vi "array_referencing.vi"() -> ()   [LabVIEW 2016]
uses:
  Type_Defs/Analog_In.ctl
panel:
  out "Array 3":u16[][](array[numeric])
  out "size(s)":i32
  out "Array 2":u16[](array[numeric])
  in  "Array":T1[](array[typedef])
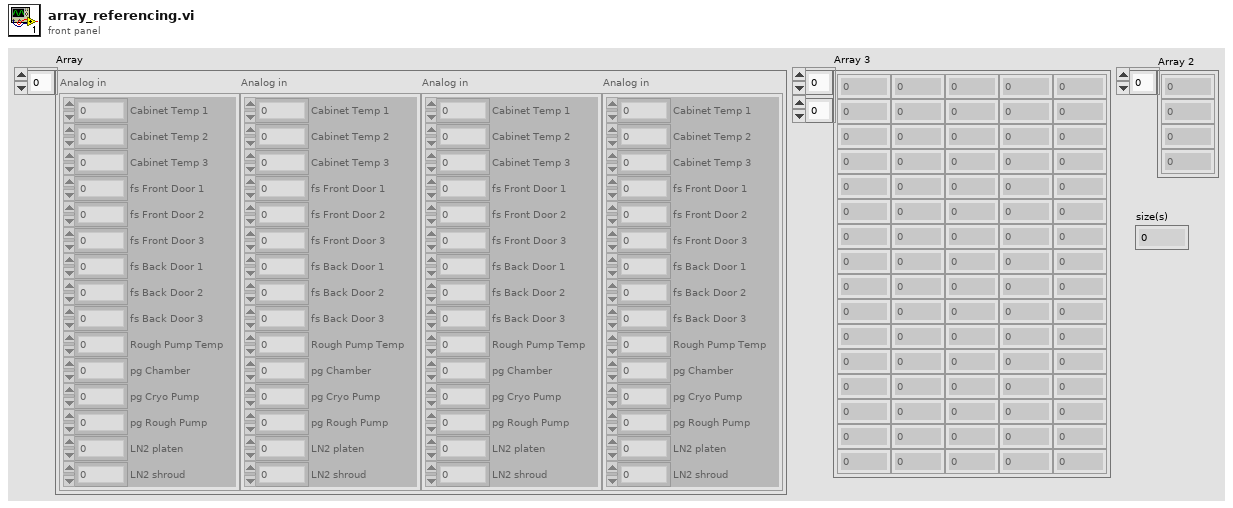
[diagram p1: front panel]
types:
  T1 = typedef "Analog_In.ctl" = cluster{"Cabinet Temp 1":u16, "Cabinet Temp 2":u16, "Cabinet Temp 3":u16, "fs Front Door 1":u16, "fs Front Door 2":u16, "fs Front Door 3":u16, "fs Back Door 1":u16, "fs Back Door 2":u16, "fs Back Door 3":u16, "Rough Pump Temp":u16, "pg Chamber":u16, "pg Cryo Pump":u16, "pg Rough Pump":u16, "LN2 platen":u16, "LN2 shroud":u16}
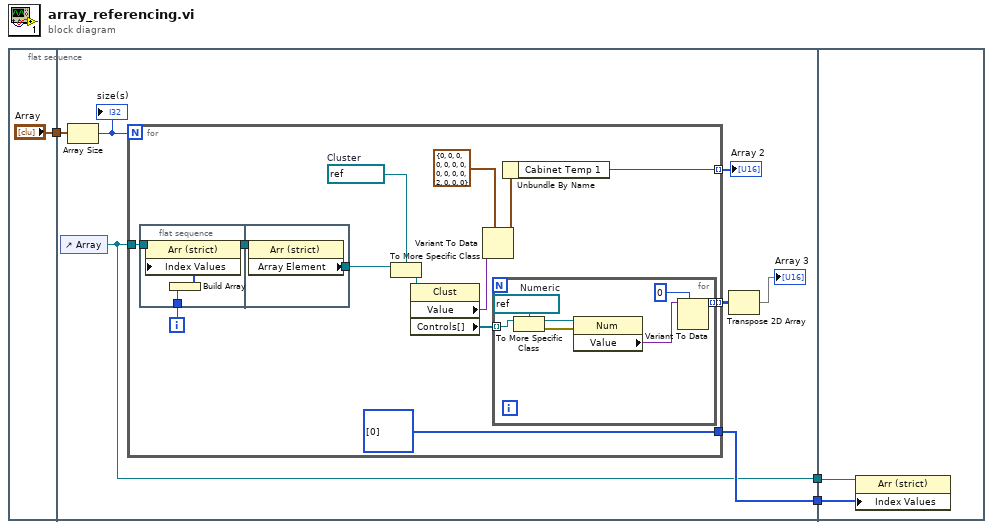
[diagram p0: block diagram]
diagram:
  n1 = flat-sequence {
    tunnel: ["Array"] -> w1
    tunnel: [w9] -> w3
    tunnel: [w8] -> w2
    tunnel: w1 -> [w5]
    tunnel: w3 -> [w38]
    tunnel: w2 -> [w39]
    frame #0 {
    }
    frame #1 {
      n2 = control-ref of="Array"() -> (w8:refnum<vi>)
      n3 = Array Size(array=w5) -> (size(s)=w11:i32)
      "size(s)" <- w11
      n4 = for {
        N: w11 -> [_]
        tunnel: w8 -> [w24]
        tunnel: [w17] -> w10 mode=indexing
        tunnel: [u32[] [0] ("Index Values")] -> w9
        tunnel: [w14] -> w7 mode=indexing
        i -> [w23]
        w19 = refnum<vi> refnum  # Cluster
        n5 = flat-sequence {
          tunnel: w24 -> [w28]
          tunnel: w23 -> [w27]
          tunnel: [w25] -> w13
          tunnel: w13 -> [w30]
          tunnel: [w29] -> w12
          frame #0 {
            n6 = Build Array(w27) -> (w26:i32[])
            n7 = property class="Arr (strict)"(reference=w28, "Index Values"=w26) -> (reference out=w25:refnum<vi>)  [unwired: 1 in, 1 out]
          }
          frame #1 {
            n8 = property class="Arr (strict)"(reference=w30) -> ("Array Element"=w29:refnum<vi>)  [unwired: 1 in, 2 out]
          }
        }
        n9 = To More Specific Class(target class=w19, reference=w12) -> (specific class reference=w20:refnum<vi>)  [unwired: 1 in, 1 out]
        n10 = property class="Clust"(reference=w20) -> ("Value"=w22:variant, "Controls[]"=w15:refnum<vi>[])  [unwired: 1 in, 2 out]
        n11 = Variant To Data(type=T1 {"Cabinet Temp 1"=0, "Cabinet Temp 2"=0, "Cabinet Temp 3"=0, "fs Front Door 1"=0, "fs Front Door 2"=0, "fs Front Door 3"=0, "fs Back Door 1"=0, "fs Back Door 2"=0, "fs Back Door 3"=0, "Rough Pump Temp"=0, "pg Chamber"=0, "pg Cryo Pump"=2, "pg Rough Pump"=0, "LN2 platen"=0, "LN2 shroud"=0} ("Analog in 2"), Variant=w22) -> (data=w18:T1)  [unwired: 1 in, 1 out]
        n12 = for {
          tunnel: w15 -> [w37] mode=indexing
          tunnel: [w31] -> w14 mode=indexing
          w36 = refnum<vi> refnum  # Numeric
          n13 = To More Specific Class(target class=w36, reference=w37) -> (specific class reference=w35:refnum<vi>, error out=w34:errorcluster)  [unwired: 1 in]
          n14 = property class="Num"(reference=w35, error in=w34) -> ("Value"=w32:variant)  [unwired: 2 out]
          n15 = Variant To Data(type=u16 0 ("cabinetTemp1"), Variant=w32) -> (data=w31:u16)  [unwired: 1 in, 1 out]
        }
        n16 = Unbundle By Name(w18) -> ("Cabinet Temp 1"=w17:u16)
      }
      "Array 2" <- w10
      n17 = Transpose 2D Array(2D array=w7) -> (transposed array=→"Array 3":u16[][])
    }
    frame #2 {
      n18 = property class="Arr (strict)"(reference=w39, "Index Values"=w38) -> ()  [unwired: 1 in, 2 out]
    }
  }
